vi "updateEndTime.vi"(8 "error in (no error)":errorcluster, 11 "RampEvent in":refnum<class "RampEvent.lvclass">) -> (0 "error out":errorcluster, 3 "RampEvent out":refnum<class "RampEvent.lvclass">)   [LabVIEW 2011, in "Tools.lvlib" / "Scripting.lvlib" / "RampEvent.lvclass"]
uses:
  RampEvent.lvclass
  RampEvent.lvclass/RampEvent.ctl
  ScriptEvent.lvclass
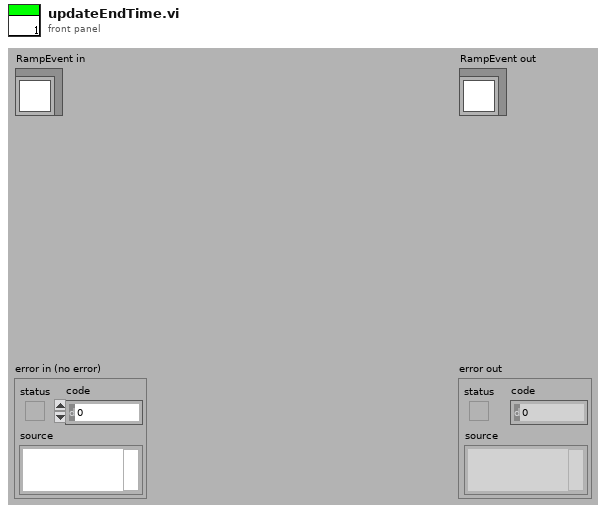
[diagram p1: front panel]
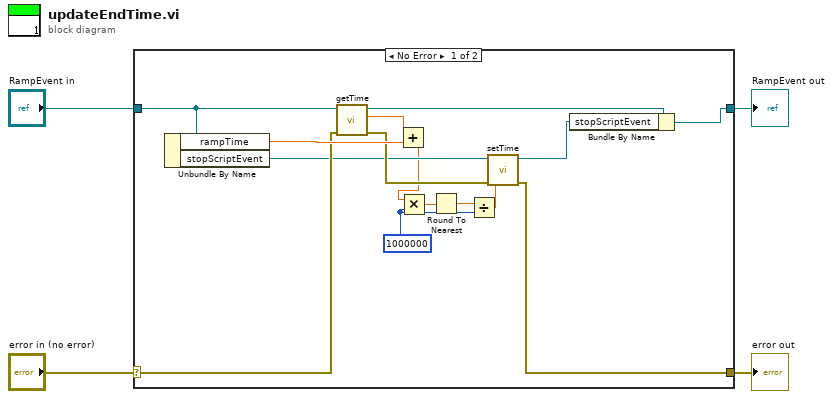
[diagram p0: block diagram]
diagram:
  n1 = case shown="No Error" "error in (no error)" {
    selector: "error in (no error)" -> [w15 w21]
    tunnel: [w11 w21] -> w3
    tunnel: [w10 w20] -> w1
    tunnel: "RampEvent in" -> [w19 w20]
    frame No Error {
      w7 = 1000000
      n2 = Unbundle By Name(w19) -> ("rampTime"=w17:dbl, "stopScriptEvent"=w14:refnum<class "ScriptEvent.lvclass">)
      n3 = call "getTime.vi"("error in (no error)"=w15, "ScriptEvent.lvclass in"=w19) -> ("error out"=w16:errorcluster, "time"=w18:dbl, "ScriptEvent.lvclass out"=w13:refnum<class "RampEvent.lvclass">)  [unwired: 7 in]
      n4 = Add(x=w18, y=w17) -> (x+y=w6:dbl)
      n5 = Multiply(x=w6, y=w7) -> (x*y=w9:dbl)
      n6 = Round To Nearest(number=w9) -> (nearest integer value=w8:dbl)
      n7 = Divide(x=w8, y=w7) -> (x/y=w5:dbl)
      n8 = call "setTime.vi"("error in (no error)"=w16, "time"=w5, "ScriptEvent.lvclass in"=w14) -> ("error out"=w11:errorcluster, "ScriptEvent.lvclass out"=w12:refnum<class "ScriptEvent.lvclass">)  [unwired: 7 in]
      n9 = Bundle By Name(cluster=w13, "stopScriptEvent"=w12) -> (w10:refnum<class "RampEvent.lvclass">)
    }
    frame Error {
    }
  }
  "error out" <- w3
  "RampEvent out" <- w1
